vi "TTA_MATLAB_Load_Settings.vi"(0 "Instruments/Criteria Settings File":path, 5 "error in":errorcluster) -> (7 "Tx Output Power Criteria Cluster":T4, 8 "Complete Settings Cluster":T1, 9 "Rx Output Power Criteria Cluster":T2, 10 "TxOffset Cal Cluster":T10, 11 "Power Cal Cluster":T6, 12 "RxOffset Cal Cluster":T9, 13 "Tx ACPR Settings Cluster":T7, 14 "Brief Cluster":T13, 15 "PAL Calibration\nInputs Cluster":T11, 16 "TX Output Power Settings Cluster":T8, 17 "Rx Received Power Settings Cluster":T5, 18 "Instrument Setting Cluster":T12, 19 "error out":errorcluster)   [LabVIEW 2016]
uses:
  TTA_Controls/TTA_Control_Complete_Settings_Cluster.ctl
  TTA_Globals/Test_Environment.vi
panel:
  out "Tx ACPR Criteria Cluster":T3
  out "Error Range Cluster":cluster{dbl, dbl, dbl, dbl, dbl, dbl}
  out "Cal Turns Cluster":cluster{dbl, dbl, dbl, dbl, dbl}
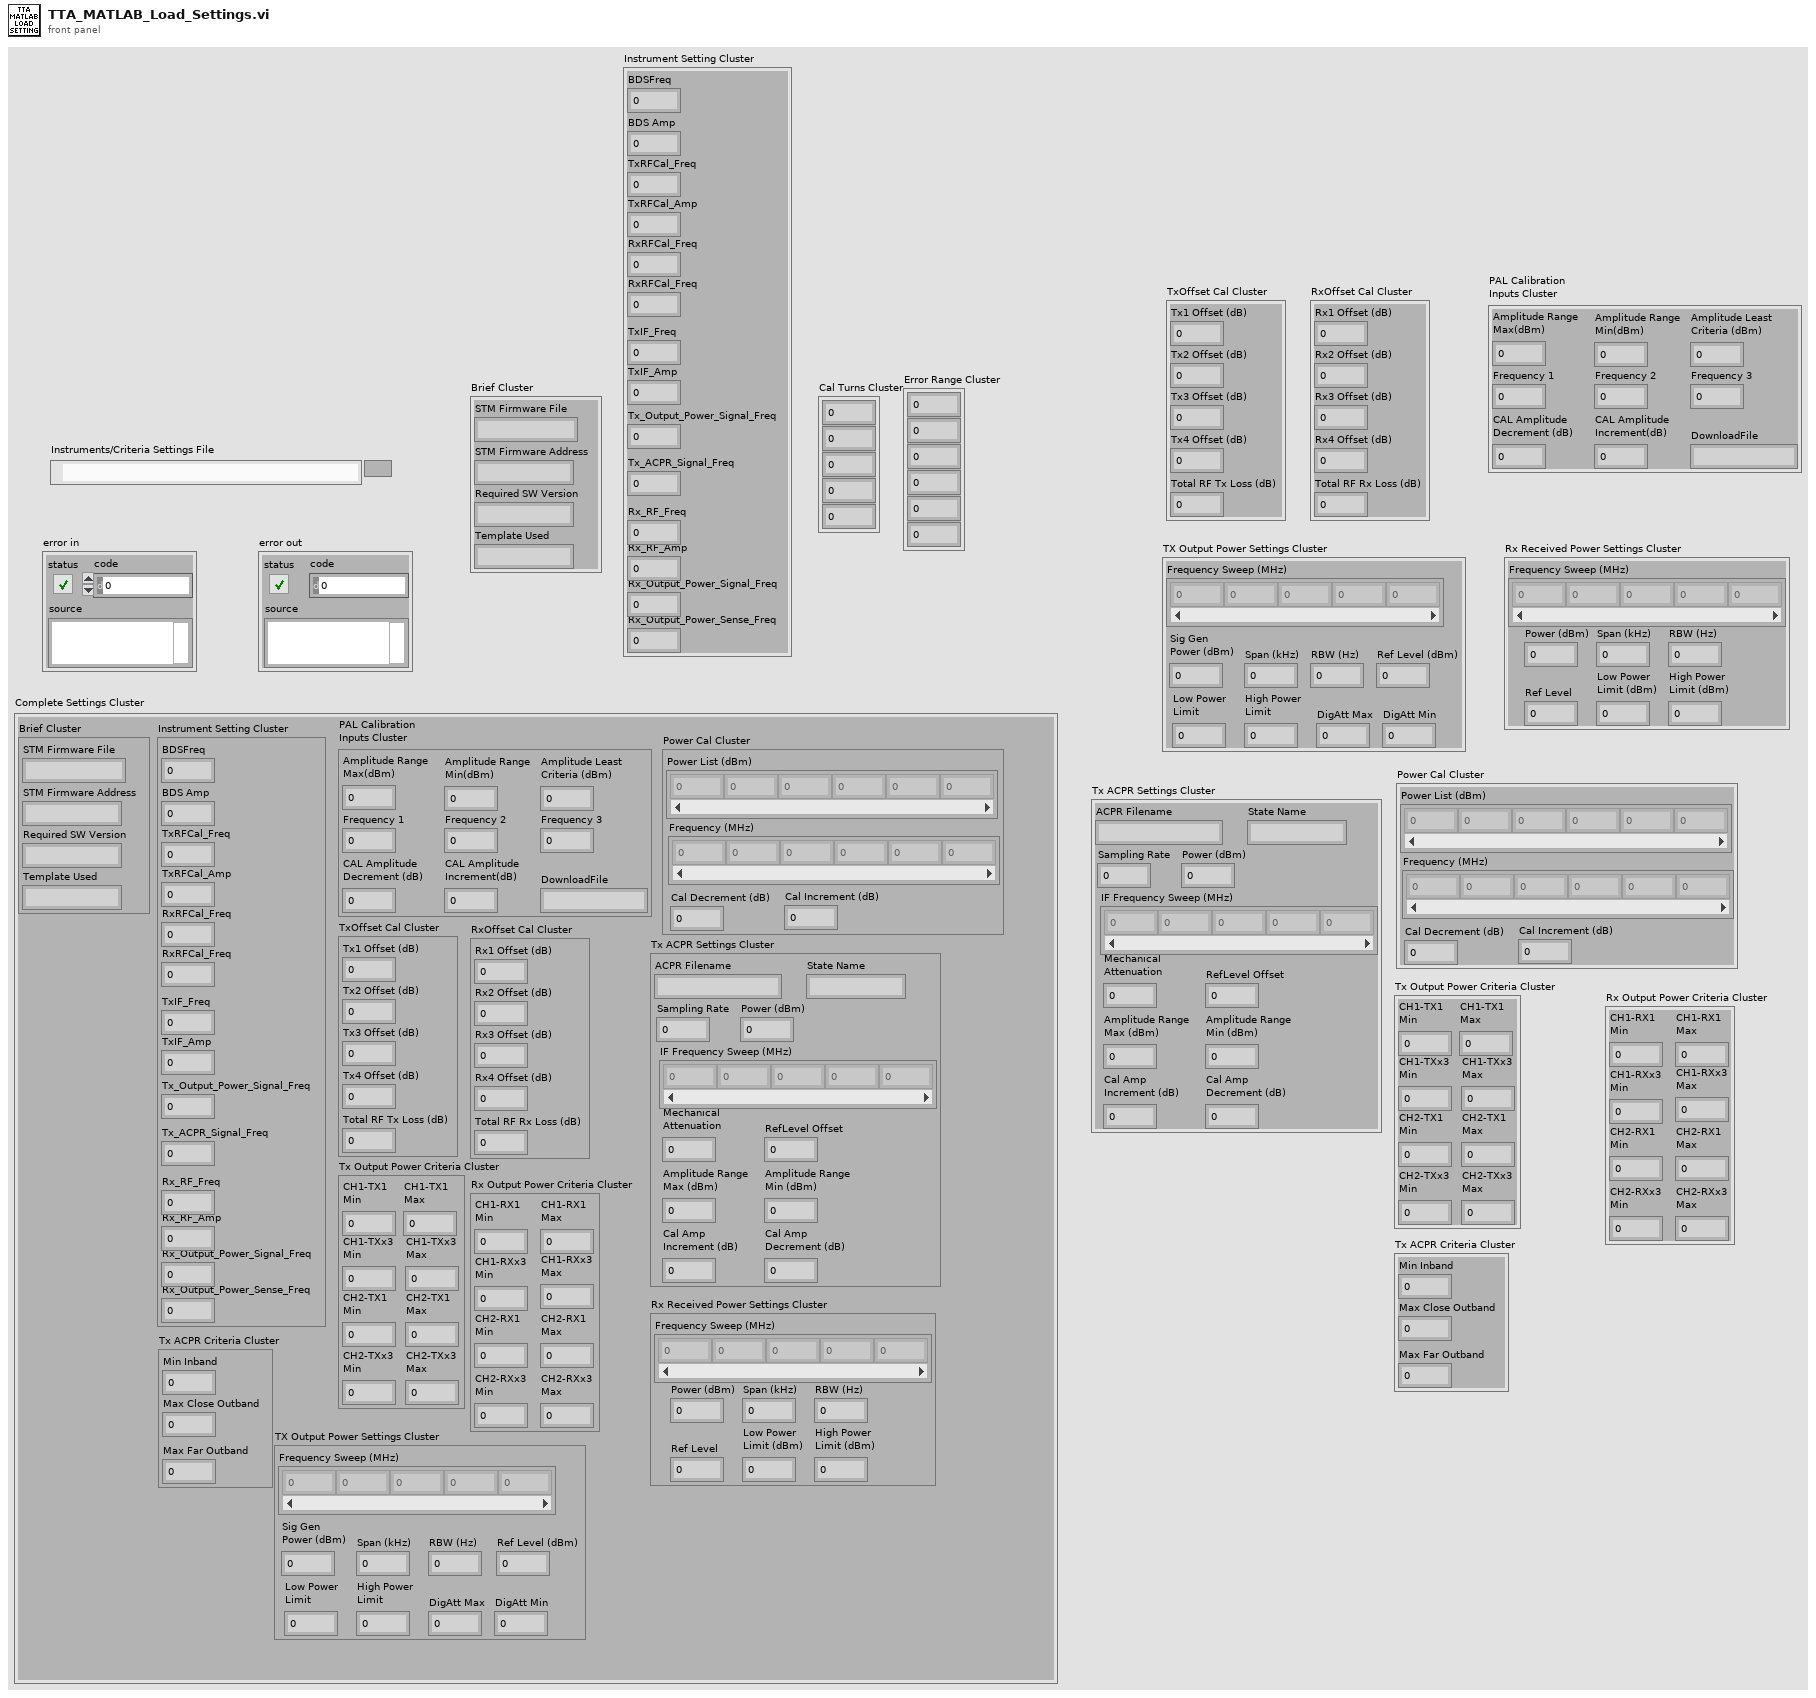
[diagram p1: front panel]
types:
  T1 = typedef "TTA_Control_Complete_Settings_Cluster.ctl" = cluster{"Brief Cluster":cluster{"STM Firmware File":string, "STM Firmware Address":string, "Required SW Version":string, "Template Used":string}, "Instrument Setting Cluster":cluster{"BDSFreq":dbl, "BDS Amp":dbl, "TxRFCal_Freq":dbl, "TxRFCal_Amp":dbl, "RxRFCal_Freq":dbl, "RxRFCal_Freq":dbl, "TxIF_Freq":dbl, "TxIF_Amp":dbl, "Tx_Output_Power_Signal_Freq":dbl, "Tx_ACPR_Signal_Freq":dbl, "Rx_RF_Freq":dbl, "Rx_RF_Amp":dbl, "Rx_Output_Power_Signal_Freq":dbl, "Rx_Output_Power_Sense_Freq":dbl}, "PAL Calibration\nInputs Cluster":cluster{"Amplitude Range\nMax(dBm)":dbl, "Amplitude Range\nMin(dBm)":dbl, "Amplitude Least\nCriteria (dBm)":dbl, "Frequency 1":dbl, "Frequency 2":dbl, "Frequency 3":dbl, "CAL Amplitude\nDecrement (dB)":dbl, "CAL Amplitude\nIncrement(dB)":dbl, "DownloadFile":string}, "TxOffset Cal Cluster":cluster{"Tx1 Offset (dB)":dbl, "Tx2 Offset (dB)":dbl, "Tx3 Offset (dB)":dbl, "Tx4 Offset (dB)":dbl, "Total RF Tx Loss (dB)":dbl}, "RxOffset Cal Cluster":cluster{"Rx1 Offset (dB)":dbl, "Rx2 Offset (dB)":dbl, "Rx3 Offset (dB)":dbl, "Rx4 Offset (dB)":dbl, "Total RF Rx Loss (dB)":dbl}, "TX Output Power Settings Cluster":cluster{"Frequency Sweep (MHz)":dbl[], "Sig Gen \nPower (dBm)":dbl, "Span (kHz)":dbl, "RBW (Hz)":dbl, "Ref Level (dBm)":dbl, "Low Power \nLimit":dbl, "High Power \nLimit":dbl, "DigAtt Max":dbl, "DigAtt Min":dbl}, "Tx ACPR Settings Cluster":cluster{"ACPR Filename":string, "Sampling Rate":dbl, "Power (dBm)":dbl, "IF Frequency Sweep (MHz)":dbl[], "State Name":string, "Mechanical\nAttenuation":dbl, "RefLevel Offset":dbl, "Amplitude Range\nMax (dBm)":dbl, "Amplitude Range\nMin (dBm)":dbl, "Cal Amp \nIncrement (dB)":dbl, "Cal Amp\nDecrement (dB)":dbl}, "Power Cal Cluster":cluster{"Power List (dBm)":dbl[], "Frequency (MHz)":dbl[], "Cal Decrement (dB)":dbl, "Cal Increment (dB)":dbl}, "Rx Received Power Settings Cluster":cluster{"Frequency Sweep (MHz)":dbl[], "Power (dBm)":dbl, "Span (kHz)":dbl, "RBW (Hz)":dbl, "Ref Level":dbl, "Low Power \nLimit (dBm)":dbl, "High Power\nLimit (dBm)":dbl}, "Tx Output Power Criteria Cluster":cluster{"CH1-TX1 \nMin":dbl, "CH1-TX1\nMax":dbl, "CH1-TXx3\nMin ":dbl, "CH1-TXx3\nMax":dbl, "CH2-TX1\nMin":dbl, "CH2-TX1\nMax":dbl, "CH2-TXx3\nMin":dbl, "CH2-TXx3\nMax":dbl}, "Tx ACPR Criteria Cluster":cluster{"Min Inband":dbl, "Max Close Outband":dbl, "Max Far Outband":dbl}, "Rx Output Power Criteria Cluster":cluster{"CH1-RX1 \nMin":dbl, "CH1-RX1 \nMax":dbl, "CH1-RXx3 \nMin":dbl, "CH1-RXx3\nMax":dbl, "CH2-RX1\nMin":dbl, "CH2-RX1\nMax":dbl, "CH2-RXx3\nMin":dbl, "CH2-RXx3\nMax":dbl}}
  T2 = cluster{"CH1-RX1 \nMin":dbl, "CH1-RX1 \nMax":dbl, "CH1-RXx3 \nMin":dbl, "CH1-RXx3\nMax":dbl, "CH2-RX1\nMin":dbl, "CH2-RX1\nMax":dbl, "CH2-RXx3\nMin":dbl, "CH2-RXx3\nMax":dbl}
  T3 = cluster{"Min Inband":dbl, "Max Close Outband":dbl, "Max Far Outband":dbl}
  T4 = cluster{"CH1-TX1 \nMin":dbl, "CH1-TX1\nMax":dbl, "CH1-TXx3\nMin ":dbl, "CH1-TXx3\nMax":dbl, "CH2-TX1\nMin":dbl, "CH2-TX1\nMax":dbl, "CH2-TXx3\nMin":dbl, "CH2-TXx3\nMax":dbl}
  T5 = cluster{"Frequency Sweep (MHz)":dbl[], "Power (dBm)":dbl, "Span (kHz)":dbl, "RBW (Hz)":dbl, "Ref Level":dbl, "Low Power \nLimit (dBm)":dbl, "High Power\nLimit (dBm)":dbl}
  T6 = cluster{"Power List (dBm)":dbl[], "Frequency (MHz)":dbl[], "Cal Decrement (dB)":dbl, "Cal Increment (dB)":dbl}
  T7 = cluster{"ACPR Filename":string, "Sampling Rate":dbl, "Power (dBm)":dbl, "IF Frequency Sweep (MHz)":dbl[], "State Name":string, "Mechanical\nAttenuation":dbl, "RefLevel Offset":dbl, "Amplitude Range\nMax (dBm)":dbl, "Amplitude Range\nMin (dBm)":dbl, "Cal Amp \nIncrement (dB)":dbl, "Cal Amp\nDecrement (dB)":dbl}
  T8 = cluster{"Frequency Sweep (MHz)":dbl[], "Sig Gen \nPower (dBm)":dbl, "Span (kHz)":dbl, "RBW (Hz)":dbl, "Ref Level (dBm)":dbl, "Low Power \nLimit":dbl, "High Power \nLimit":dbl, "DigAtt Max":dbl, "DigAtt Min":dbl}
  T9 = cluster{"Rx1 Offset (dB)":dbl, "Rx2 Offset (dB)":dbl, "Rx3 Offset (dB)":dbl, "Rx4 Offset (dB)":dbl, "Total RF Rx Loss (dB)":dbl}
  T10 = cluster{"Tx1 Offset (dB)":dbl, "Tx2 Offset (dB)":dbl, "Tx3 Offset (dB)":dbl, "Tx4 Offset (dB)":dbl, "Total RF Tx Loss (dB)":dbl}
  T11 = cluster{"Amplitude Range\nMax(dBm)":dbl, "Amplitude Range\nMin(dBm)":dbl, "Amplitude Least\nCriteria (dBm)":dbl, "Frequency 1":dbl, "Frequency 2":dbl, "Frequency 3":dbl, "CAL Amplitude\nDecrement (dB)":dbl, "CAL Amplitude\nIncrement(dB)":dbl, "DownloadFile":string}
  T12 = cluster{"BDSFreq":dbl, "BDS Amp":dbl, "TxRFCal_Freq":dbl, "TxRFCal_Amp":dbl, "RxRFCal_Freq":dbl, "RxRFCal_Freq":dbl, "TxIF_Freq":dbl, "TxIF_Amp":dbl, "Tx_Output_Power_Signal_Freq":dbl, "Tx_ACPR_Signal_Freq":dbl, "Rx_RF_Freq":dbl, "Rx_RF_Amp":dbl, "Rx_Output_Power_Signal_Freq":dbl, "Rx_Output_Power_Sense_Freq":dbl}
  T13 = cluster{"STM Firmware File":string, "STM Firmware Address":string, "Required SW Version":string, "Template Used":string}
  T14 = cluster{dbl, dbl, dbl, dbl, dbl, dbl, dbl, dbl, string}
  T15 = cluster{dbl[], dbl, dbl, dbl, dbl, dbl, dbl, dbl, dbl}
  T16 = cluster{string, dbl, dbl, dbl[], string, dbl, dbl, dbl, dbl, dbl, dbl}
  T17 = cluster{dbl, dbl, dbl, dbl, dbl, dbl, dbl, dbl, dbl, dbl, dbl, dbl, dbl, dbl}
  T18 = cluster{cluster{string, string, string, string}, cluster{dbl, dbl, dbl, dbl, dbl, dbl, dbl, dbl, dbl, dbl, dbl, dbl, dbl, dbl}, cluster{dbl, dbl, dbl, dbl, dbl, dbl, dbl, dbl, string}, cluster{dbl, dbl, dbl, dbl, dbl}, cluster{dbl, dbl, dbl, dbl, dbl}, cluster{dbl[], dbl, dbl, dbl, dbl, dbl, dbl, dbl, dbl}, cluster{string, dbl, dbl, dbl[], string, dbl, dbl, dbl, dbl, dbl, dbl}, cluster{dbl[], dbl[], dbl, dbl}, cluster{dbl[], dbl, dbl, dbl, dbl, dbl, dbl}, cluster{dbl, dbl, dbl, dbl, dbl, dbl, dbl, dbl}, cluster{dbl, dbl, dbl}, cluster{dbl, dbl, dbl, dbl, dbl, dbl, dbl, dbl}}
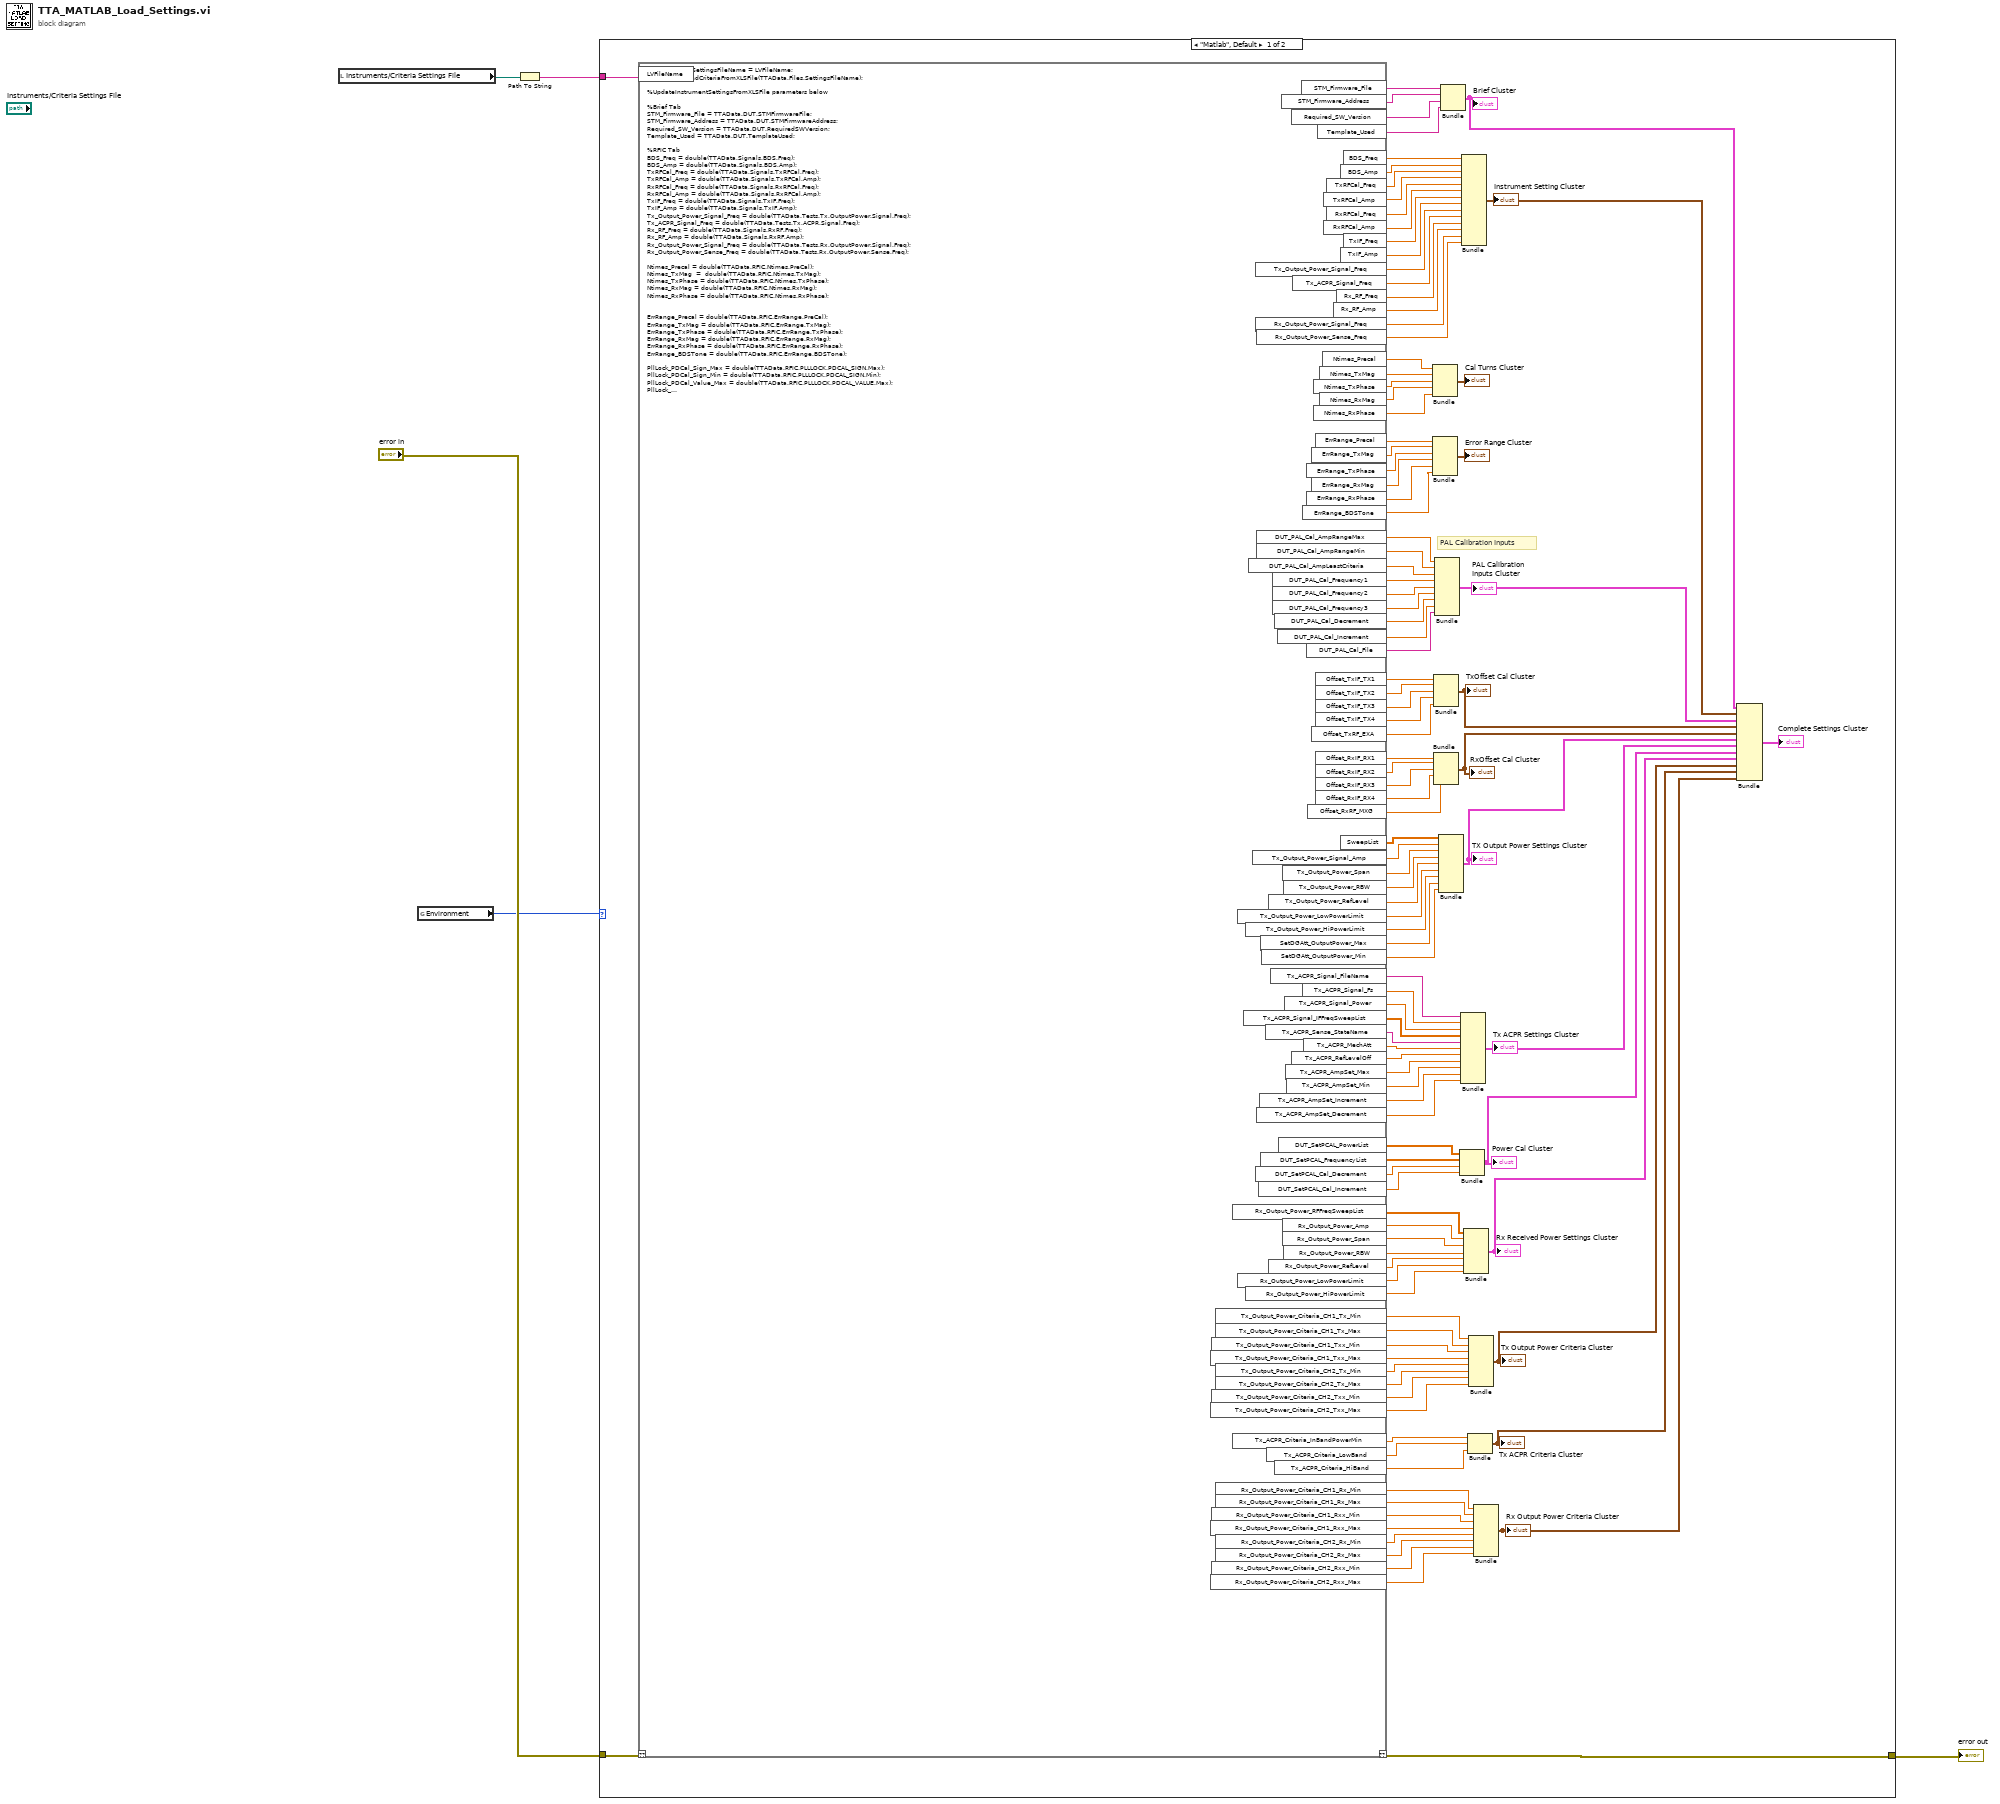
[diagram p0: block diagram]
diagram:
  n1 = local read "Instruments/Criteria Settings File"() -> (w5:path)
  n2 = global read "Test_Environment.vi" "Environment"() -> (w1:enum16{"Matlab", "LabVIEW"})
  n3 = Path To String(path=w5) -> (string=w4:string)
  n4 = case shown="\"Matlab\", Default" w1 {
    tunnel: w4 -> [w121 _]
    tunnel: "error in" -> [w120 w122]
    tunnel: [w119 w122] -> w2
    frame "Matlab", Default {
      # "PAL Calibration Inputs"
      n5 = script code="TTAData.Files.SettingsFileName = LVFileName;\nLoadSettingsAndCriteriaFromXLSFile(TTAData.Files.SettingsFileName);\n\n%UpdateInstrumentSettingsFromXLSFile parameters below\n\n%Brief Tab\nSTM_Firmware_File = TTAData.DUT.STMFirmwareFile;\nSTM_Firmware_Address = TTAData.DUT.STMFirmwareAddress;\nRequired_SW_Version = TTAData.DUT.RequiredSWVersion;\nTemplate_Used = TTAData.DUT.TemplateUsed;\n\n%RFIC Tab\nBDS_Freq = double(TTAData.Signals.BDS.Freq);\nBDS_Amp = double(TTAData.Signals.BDS.Amp);\nTxRFCal_Freq = double(TTAData.Signals.TxRFCal.Freq);\nTxRFCal_Amp = double(TTAData.Signals.TxRFCal.Amp);\nRxRFCal_Freq = double(TTAData.Signals.RxRFCal.Freq);\nRxRFCal_Amp = double(TTAData.Signals.RxRFCal.Amp);\nTxIF_Freq = double(TTAData.Signals.TxIF.Freq);\nTxIF_Amp = double(TTAData.Signals.TxIF.Amp);\nTx_Output_Power_Signal_Freq = double(TTAData.Tests.Tx.OutputPower.Signal.Freq);\nTx_ACPR_Signal_Freq = double(TTAData.Tests.Tx.ACPR.Signal.Freq);\nRx_RF_Freq = double(TTAData.Signals.RxRF.Freq);\nRx_RF_Amp = double(TTAData.Signals.RxRF.Amp);\nRx_Output_Power_Signal_Freq = double(TTAData.Tests.Rx.OutputPower.Signal.Freq);\nRx_Output_Power_Sense_Freq = double(TTAData.Tests.Rx.OutputPower.Sense.Freq);\n\nNtimes_Precal = double(TTAData.RFIC.Ntimes.PreCal);\nNtimes_TxMag  =  double(TTAData.RFIC.Ntimes.TxMag);\nNtimes_TxPhase = double(TTAData.RFIC.Ntimes.TxPhase);\nNtimes_RxMag = double(TTAData.RFIC.Ntimes.RxMag);\nNtimes_RxPhase = double(TTAData.RFIC.Ntimes.RxPhase);\n\n\nErrRange_Precal = double(TTAData.RFIC.ErrRange.PreCal);\nErrRange_TxMag = double(TTAData.RFIC.ErrRange.TxMag);\nErrRange_TxPhase = double(TTAData.RFIC.ErrRange.TxPhase);\nErrRange_RxMag = double(TTAData.RFIC.ErrRange.RxMag);\nErrRange_RxPhase = double(TTAData.RFIC.ErrRange.RxPhase);\nErrRange_BDSTone = double(TTAData.RFIC.ErrRange.BDSTone);\n\nPllLock_PDCal_Sign_Max = double(TTAData.RFIC.PLLLOCK.PDCAL_SIGN.Max); \nPllLock_PDCal_Sign_Min = double(TTAData.RFIC.PLLLOCK.PDCAL_SIGN.Min);\nPllLock_PDCal_Value_Max = double(TTAData.RFIC.PLLLOCK.PDCAL_VALUE.Max);\nPllLock_PDCal_Value_Min = double(TTAData.RFIC.PLLLOCK.PDCAL_VALUE.Min);\nPllLock_Bcal_Max = double(TTAData.RFIC.PLLLOCK.BCAL.Max);\nPllLock_Bcal_Min = double(TTAData.RFIC.PLLLOCK.BCAL.Min);\nRFCal_MagCal_Max = double(TTAData.RFIC.RFCAL.MAGCAL.Max);\nRFCal_MagCal_Min = double(TTAData.RFIC.RFCAL.MAGCAL.Min);\nRFCal_PhCal_Max = double(TTAData.RFIC.RFCAL.PHCAL.Max);\nRFCal_PhCal_Min = double(TTAData.RFIC.RFCAL.PHCAL.Min);\nRF_Cal_PreCal_PdCal_Sign_Max = double(TTAData.RFIC.RFCAL.PRECAL.PDCAL_SIGN.Max);\nRF_Cal_PreCal_PdCal_Sign_Min = double(TTAData.RFIC.RFCAL.PRECAL.PDCAL_SIGN.Min);\nRF_Cal_PreCal_PdCal_Value_Max = double(TTAData.RFIC.RFCAL.PRECAL.PDCAL_VALUE.Max);\nRF_Cal_PreCal_PdCal_Value_Min = double(TTAData.RFIC.RFCAL.PRECAL.PDCAL_VALUE.Min);\nRF_Cal_PllLock_BCal_Max = double(TTAData.RFIC.RFCAL.PLLLOCK.BCAL_Max);\nRF_Cal_PllLock_BCal_Min = double(TTAData.RFIC.RFCAL.PLLLOCK.BCAL_Min);\nRFIC_Temp_Max = double(TTAData.RFIC.TEMP.Max);\nRFIC_Temp_Min = double(TTAData.RFIC.TEMP.Min);\nRFIC_RFCal_Mode_CoarseOnly = double(TTAData.RFIC.RFCAL.MODE.COARSEONLY);\nRFIC_RFCal_Mode_ExtFineStop = double(TTAData.RFIC.RFCAL.MODE.EXTFINESTOP);\nRFIC_RFCal_Mode_Att = double(TTAData.RFIC.RFCAL.MODE.ATT);\nRFIC_RFCal_Mode_PreDist = double(TTAData.RFIC.RFCAL.MODE.PREDIST);\nRFIC_RFCal_Mode_Deg180Fix = double(TTAData.RFIC.RFCAL.MODE.DEG180FIX);\nRFIC_RFCal_Mode_PAOutPwrLoop = double(TTAData.RFIC.RFCAL.MODE.PAOUTPWRLOOP);\nRFIC_RFCal_Mode_PAInPwrLoop = double(TTAData.RFIC.RFCAL.MODE.PAINPWRLOOP);\nRFIC_RFCal_Mode_PABias_Loop = double(TTAData.RFIC.RFCAL.MODE.PABIASLOOP);\nRFIC_RFCal_Att_Temp_Nom = double(TTAData.RFIC.RFCAL.ATT.TEMP_NOM);\nRFIC_RFCal_Att_Slope = double(TTAData.RFIC.RFCAL.ATT.SLOPE);\nRFIC_RFCal_DelayFine = double(TTAData.RFIC.RFCAL.DELAYFINE);\nRFIC_RFCal_TxAmpGain = double(TTAData.RFIC.RFCAL.TXAMPGAIN);\nRFIC_RFCal_Nom_Offset_MagTx = double(TTAData.RFIC.RFCAL.NOM_OFFSET_MAGTX);\nRFIC_RFCal_RxAmpGain =     double(TTAData.RFIC.RFCAL.RXAMPGAIN);\n\nRFIC_RFCal_Delay_RxRFCal = double(TTAData.RFIC.RFCAL.DELAY_RxRFCAL);\n\nRFIC_Nom_Mag_Tx = double(TTAData.RFIC.NOM_MAG_TX);\nRFIC_Nom_Mag_Rx = double(TTAData.RFIC.NOM_MAG_RX);\nRFIC_MagLUT = double(TTAData.RFIC.MAGLUT);\nRFIC_PhLUT = double(TTAData.RFIC.PHLUT);\nRFIC_Resample = double(TTAData.RFIC.RESAMPLE);\nRFIC_RFCal_DelayCourse = double(TTAData.RFIC.RFCAL.DELAYCOARSE);\n\n%*****************Tx ACPR Tab**********************\nDUT_PAL_Cal_AmpRangeMax = double(TTAData.DUT.PAL_CAL.AmpRangeMax);\nDUT_PAL_Cal_AmpRangeMin = double(TTAData.DUT.PAL_CAL.AmpRangeMin);\nDUT_PAL_Cal_AmpLeastCriteria = double(TTAData.DUT.PAL_CAL.AmpLeastCriteria);\nDUT_PAL_Cal_Frequency1 = double(TTAData.DUT.PAL_CAL.Frequency1);\nDUT_PAL_Cal_Frequency2 = double(TTAData.DUT.PAL_CAL.Frequency2);\nDUT_PAL_Cal_Frequency3 = double(TTAData.DUT.PAL_CAL.Frequency3);\nDUT_PAL_Cal_Decrement = double(TTAData.DUT.PAL_CAL.CAL_Decrement);\nDUT_PAL_Cal_Increment = double(TTAData.DUT.PAL_CAL.CAL_Increment);\nDUT_PAL_Cal_File = char(TTAData.DUT.PAL_CAL.DownloadFile);\n\nTx_ACPR_Signal_FileName = char(TTAData.Tests.Tx.ACPR.Signal.FileName);\nTx_ACPR_Signal_Fs = double(TTAData.Tests.Tx.ACPR.Signal.Fs);\nTx_ACPR_Signal_Power = double(TTAData.Tests.Tx.ACPR.Signal.Power);\nTx_ACPR_Signal_IFFreqSweepList = double(TTAData.Tests.Tx.ACPR.Signal.IFFreqSweepList);\nTx_ACPR_Sense_StateName = char(TTAData.Tests.Tx.ACPR.Sense.StateName);\nTx_ACPR_MechAtt = double(TTAData.Tests.Tx.ACPR.MechAtt);\nTx_ACPR_RefLevelOff = double(TTAData.Tests.Tx.ACPR.RefLevelOff);\nTx_ACPR_AmpSet_Max = double(TTAData.Tests.Tx.ACPR.AmpSet.Max);\nTx_ACPR_AmpSet_Min = double(TTAData.Tests.Tx.ACPR.AmpSet.Min);\nTx_ACPR_AmpSet_Increment = double(TTAData.Tests.Tx.ACPR.AmpSet.Increment);\nTx_ACPR_AmpSet_Decrement = double(TTAData.Tests.Tx.ACPR.AmpSet.Decrement);\n\n%*****************TxRxOffset CAL Tab**********************\nOffset_TxIF_TX1 = double(TTAData.Offset.TxIF.TX1);\nOffset_TxIF_TX2 = double(TTAData.Offset.TxIF.TX2);\nOffset_TxIF_TX3 = double(TTAData.Offset.TxIF.TX3);\nOffset_TxIF_TX4 = double(TTAData.Offset.TxIF.TX4);\nOffset_TxIF_TXx3 = double(TTAData.Offset.TxIF.TXx3);\nOffset_TxIF_TXx4 = double(TTAData.Offset.TxIF.TXx4);\nOffset_TxRF_EXA = double(TTAData.Offset.TxRF.EXA);\n\nOffset_RxIF_RX1 = double(TTAData.Offset.RxIF.RX1);\nOffset_RxIF_RX2 = double(TTAData.Offset.RxIF.RX2);\nOffset_RxIF_RX3 = double(TTAData.Offset.RxIF.RX3);\nOffset_RxIF_RX4 = double(TTAData.Offset.RxIF.RX4);\nOffset_RxIF_RXx3 = double(TTAData.Offset.RxIF.RXx3);\nOffset_RxIF_RXx4 = double(TTAData.Offset.RxIF.RXx4);\nOffset_RxRF_MXG = double(TTAData.Offset.RxRF.MXG);\n\n%*****************Tx Output Power Tab**********************\nSweepList = double(TTAData.Tests.Tx.OutputPower.Signal.IFFreqSweepList);\nTx_Output_Power_Signal_Amp = double(TTAData.Tests.Tx.OutputPower.Signal.Amp);;\nTx_Output_Power_Span = double(TTAData.Tests.Tx.OutputPower.Sense.Span);\nTx_Output_Power_RBW = double(TTAData.Tests.Tx.OutputPower.Sense.RBW);\nTx_Output_Power_RefLevel = double(TTAData.Tests.Tx.OutputPower.Sense.RefLevel);\nTx_Output_Power_LowPowerLimit= double(TTAData.Tests.Tx.OutputPower.Sense.LowPowerLimit);\nTx_Output_Power_HiPowerLimit = double(TTAData.Tests.Tx.OutputPower.Sense.HiPowerLimit);\nSetDGAtt_OutputPower_Max = double(TTAData.SetDGAtt.OutputPower.Max);\nSetDGAtt_OutputPower_Min = double(TTAData.SetDGAtt.OutputPower.Min);\n\n%*****************Power Cal Tab**********************\nDUT_SetPCAL_PowerList = double(TTAData.DUT.SetPCAL.PowerList);\nDUT_SetPCAL_FrequencyList = double(TTAData.DUT.SetPCAL.Frequency);\nDUT_SetPCAL_Cal_Decrement = double(TTAData.DUT.SetPCAL.CAL_Decrement);\nDUT_SetPCAL_Cal_Increment = double(TTAData.DUT.SetPCAL.CAL_Increment);\n\n%*****************Rx Received Power Tab**********************\nRx_Output_Power_RFFreqSweepList = double(TTAData.Tests.Rx.OutputPower.Signal.RFFreqSweepList);\nRx_Output_Power_Amp = double(TTAData.Tests.Rx.OutputPower.Signal.Amp);\nRx_Output_Power_Span = double(TTAData.Tests.Rx.OutputPower.Sense.Span);\nRx_Output_Power_RBW = double(TTAData.Tests.Rx.OutputPower.Sense.RBW);\nRx_Output_Power_RefLevel = double(TTAData.Tests.Rx.OutputPower.Sense.RefLevel);\nRx_Output_Power_LowPowerLimit = double(TTAData.Tests.Rx.OutputPower.Sense.LowPowerLimit);\nRx_Output_Power_HiPowerLimit = double(TTAData.Tests.Rx.OutputPower.Sense.HiPowerLimit);\n\n\n%*****************Tx Output Power Criteria**********************\nTx_Output_Power_Criteria_CH1_Tx_Min = double(TTAData.Tests.Tx.OutputPower.Criteria.CH1Tx.MinIFAmp);\nTx_Output_Power_Criteria_CH1_Tx_Max = double(TTAData.Tests.Tx.OutputPower.Criteria.CH1Tx.MaxIFAmp);\nTx_Output_Power_Criteria_CH1_Txx_Min = double(TTAData.Tests.Tx.OutputPower.Criteria.CH1Txx.MinIFAmp);\nTx_Output_Power_Criteria_CH1_Txx_Max = double(TTAData.Tests.Tx.OutputPower.Criteria.CH1Txx.MaxIFAmp);\nTx_Output_Power_Criteria_CH2_Tx_Min = double(TTAData.Tests.Tx.OutputPower.Criteria.CH2Tx.MinIFAmp);\nTx_Output_Power_Criteria_CH2_Tx_Max = double(TTAData.Tests.Tx.OutputPower.Criteria.CH2Tx.MaxIFAmp);\nTx_Output_Power_Criteria_CH2_Txx_Min = double(TTAData.Tests.Tx.OutputPower.Criteria.CH2Txx.MinIFAmp);\nTx_Output_Power_Criteria_CH2_Txx_Max = double(TTAData.Tests.Tx.OutputPower.Criteria.CH2Txx.MaxIFAmp);\n\n%*****************Tx ACPR Criteria**********************\nTx_ACPR_Criteria_InBandPowerMin = double(TTAData.Tests.Tx.ACPR.Criteria.InBandPowerMin);\nTx_ACPR_Criteria_LowBand = double(TTAData.Tests.Tx.ACPR.Criteria.ACPRLowBand);\nTx_ACPR_Criteria_HiBand = double(TTAData.Tests.Tx.ACPR.Criteria.ACPRHiBand);\n\n%*****************Rx Received Power Criteria**********************\nRx_Output_Power_Criteria_CH1_Rx_Min = double(TTAData.Tests.Rx.OutputPower.Criteria.CH1Rx.MinIFAmp);\nRx_Output_Power_Criteria_CH1_Rx_Max = double(TTAData.Tests.Rx.OutputPower.Criteria.CH1Rx.MaxIFAmp);\nRx_Output_Power_Criteria_CH1_Rxx_Min = double(TTAData.Tests.Rx.OutputPower.Criteria.CH1Rxx.MinIFAmp);\nRx_Output_Power_Criteria_CH1_Rxx_Max = double(TTAData.Tests.Rx.OutputPower.Criteria.CH1Rxx.MaxIFAmp);\nRx_Output_Power_Criteria_CH2_Rx_Min = double(TTAData.Tests.Rx.OutputPower.Criteria.CH2Rx.MinIFAmp);\nRx_Output_Power_Criteria_CH2_Rx_Max = double(TTAData.Tests.Rx.OutputPower.Criteria.CH2Rx.MaxIFAmp);\nRx_Output_Power_Criteria_CH2_Rxx_Min = double(TTAData.Tests.Rx.OutputPower.Criteria.CH2Rxx.MinIFAmp);\nRx_Output_Power_Criteria_CH2_Rxx_Max = double(TTAData.Tests.Rx.OutputPower.Criteria.CH2Rxx.MaxIFAmp);"("??"=w120, "LVFileName"=w121) -> ("??"=w119:errorcluster, "STM_Firmware_File"=w118:string, "STM_Firmware_Address"=w117:string, "Required_SW_Version"=w116:string, "Template_Used"=w115:string, "BDS_Freq"=w108:dbl, "BDS_Amp"=w107:dbl, "TxRFCal_Freq"=w106:dbl, "TxRFCal_Amp"=w105:dbl, "RxRFCal_Freq"=w104:dbl, "RxRFCal_Amp"=w103:dbl, "TxIF_Freq"=w102:dbl, "TxIF_Amp"=w101:dbl, "Tx_Output_Power_Signal_Freq"=w100:dbl, "Tx_ACPR_Signal_Freq"=w99:dbl, "Rx_RF_Freq"=w98:dbl, "Rx_RF_Amp"=w97:dbl, "Rx_Output_Power_Signal_Freq"=w96:dbl, "Rx_Output_Power_Sense_Freq"=w95:dbl, "Ntimes_Precal"=w114:dbl, "Ntimes_TxMag"=w113:dbl, "Ntimes_TxPhase"=w112:dbl, "Ntimes_RxMag"=w111:dbl, "Ntimes_RxPhase"=w110:dbl, "ErrRange_Precal"=w94:dbl, "ErrRange_TxMag"=w93:dbl, "ErrRange_TxPhase"=w92:dbl, "ErrRange_RxMag"=w91:dbl, "ErrRange_RxPhase"=w90:dbl, "ErrRange_BDSTone"=w89:dbl, "DUT_PAL_Cal_AmpRangeMax"=w87:dbl, "DUT_PAL_Cal_AmpRangeMin"=w86:dbl, "DUT_PAL_Cal_AmpLeastCriteria"=w85:dbl, "DUT_PAL_Cal_Frequency1"=w84:dbl, "DUT_PAL_Cal_Frequency2"=w83:dbl, "DUT_PAL_Cal_Frequency3"=w82:dbl, "DUT_PAL_Cal_Decrement"=w81:dbl, "DUT_PAL_Cal_Increment"=w80:dbl, "DUT_PAL_Cal_File"=w79:string, "Offset_TxIF_TX1"=w78:dbl, "Offset_TxIF_TX2"=w77:dbl, "Offset_TxIF_TX3"=w76:dbl, "Offset_TxIF_TX4"=w75:dbl, "Offset_TxRF_EXA"=w74:dbl, "Offset_RxIF_RX1"=w73:dbl, "Offset_RxIF_RX2"=w72:dbl, "Offset_RxIF_RX3"=w71:dbl, "Offset_RxIF_RX4"=w70:dbl, "Offset_RxRF_MXG"=w69:dbl, "SweepList"=w7:dbl[], "Tx_Output_Power_Signal_Amp"=w8:dbl, "Tx_Output_Power_Span"=w68:dbl, "Tx_Output_Power_RBW"=w67:dbl, "Tx_Output_Power_RefLevel"=w66:dbl, "Tx_Output_Power_LowPowerLimit"=w65:dbl, "Tx_Output_Power_HiPowerLimit"=w64:dbl, "SetDGAtt_OutputPower_Max"=w63:dbl, "SetDGAtt_OutputPower_Min"=w62:dbl, "Tx_ACPR_Signal_FileName"=w51:string, "Tx_ACPR_Signal_Fs"=w52:dbl, "Tx_ACPR_Signal_Power"=w53:dbl, "Tx_ACPR_Signal_IFFreqSweepList"=w61:dbl[], "Tx_ACPR_Sense_StateName"=w60:string, "Tx_ACPR_MechAtt"=w59:dbl, "Tx_ACPR_RefLevelOff"=w58:dbl, "Tx_ACPR_AmpSet_Max"=w57:dbl, "Tx_ACPR_AmpSet_Min"=w56:dbl, "Tx_ACPR_AmpSet_Increment"=w55:dbl, "Tx_ACPR_AmpSet_Decrement"=w54:dbl, "DUT_SetPCAL_PowerList"=w50:dbl[], "DUT_SetPCAL_FrequencyList"=w49:dbl[], "DUT_SetPCAL_Cal_Decrement"=w48:dbl, "DUT_SetPCAL_Cal_Increment"=w47:dbl, "Rx_Output_Power_RFFreqSweepList"=w46:dbl[], "Rx_Output_Power_Amp"=w45:dbl, "Rx_Output_Power_Span"=w44:dbl, "Rx_Output_Power_RBW"=w43:dbl, "Rx_Output_Power_RefLevel"=w42:dbl, "Rx_Output_Power_LowPowerLimit"=w41:dbl, "Rx_Output_Power_HiPowerLimit"=w40:dbl, "Tx_Output_Power_Criteria_CH1_Tx_Min"=w39:dbl, "Tx_Output_Power_Criteria_CH1_Tx_Max"=w38:dbl, "Tx_Output_Power_Criteria_CH1_Txx_Min"=w37:dbl, "Tx_Output_Power_Criteria_CH1_Txx_Max"=w36:dbl, "Tx_Output_Power_Criteria_CH2_Tx_Min"=w35:dbl, "Tx_Output_Power_Criteria_CH2_Tx_Max"=w34:dbl, "Tx_Output_Power_Criteria_CH2_Txx_Min"=w33:dbl, "Tx_Output_Power_Criteria_CH2_Txx_Max"=w32:dbl, "Tx_ACPR_Criteria_InBandPowerMin"=w31:dbl, "Tx_ACPR_Criteria_LowBand"=w30:dbl, "Tx_ACPR_Criteria_HiBand"=w29:dbl, "Rx_Output_Power_Criteria_CH1_Rx_Min"=w28:dbl, "Rx_Output_Power_Criteria_CH1_Rx_Max"=w27:dbl, "Rx_Output_Power_Criteria_CH1_Rxx_Min"=w26:dbl, "Rx_Output_Power_Criteria_CH1_Rxx_Max"=w25:dbl, "Rx_Output_Power_Criteria_CH2_Rx_Min"=w24:dbl, "Rx_Output_Power_Criteria_CH2_Rx_Max"=w23:dbl, "Rx_Output_Power_Criteria_CH2_Rxx_Min"=w22:dbl, "Rx_Output_Power_Criteria_CH2_Rxx_Max"=w21:dbl)
      n6 = Bundle(w114, w113, w112, w111, w110) -> (→"Cal Turns Cluster":cluster{dbl, dbl, dbl, dbl, dbl})  [unwired: 1 in]
      n7 = Bundle(w94, w93, w92, w91, w90, w89) -> (→"Error Range Cluster":cluster{dbl, dbl, dbl, dbl, dbl, dbl})  [unwired: 1 in]
      n8 = Bundle(w78, w77, w76, w75, w74) -> (w17:cluster{dbl, dbl, dbl, dbl, dbl})  [unwired: 1 in]
      "TxOffset Cal Cluster" <- w17
      n9 = Bundle(w73, w72, w71, w70, w69) -> (w16:cluster{dbl, dbl, dbl, dbl, dbl})  [unwired: 1 in]
      "RxOffset Cal Cluster" <- w16
      n10 = Bundle(w87, w86, w85, w84, w83, w82, w81, w80, w79) -> (w18:T14)  [unwired: 1 in]
      "PAL Calibration\nInputs Cluster" <- w18
      n11 = Bundle(w7, w8, w68, w67, w66, w65, w64, w63, w62) -> (w6:T15)  [unwired: 1 in]
      "TX Output Power Settings Cluster" <- w6
      n12 = Bundle(w118, w117, w116, w115) -> (w20:cluster{string, string, string, string})  [unwired: 1 in]
      "Brief Cluster" <- w20
      n13 = Bundle(w50, w49, w48, w47) -> (w14:cluster{dbl[], dbl[], dbl, dbl})  [unwired: 1 in]
      "Power Cal Cluster" <- w14
      n14 = Bundle(w51, w52, w53, w61, w60, w59, w58, w57, w56, w55, w54) -> (w15:T16)  [unwired: 1 in]
      "Tx ACPR Settings Cluster" <- w15
      n15 = Bundle(w108, w107, w106, w105, w104, w103, w102, w101, w100, w99, w98, w97, w96, w95) -> (w19:T17)  [unwired: 1 in]
      "Instrument Setting Cluster" <- w19
      n16 = Bundle(w46, w45, w44, w43, w42, w41, w40) -> (w13:cluster{dbl[], dbl, dbl, dbl, dbl, dbl, dbl})  [unwired: 1 in]
      "Rx Received Power Settings Cluster" <- w13
      n17 = Bundle(w31, w30, w29) -> (w11:cluster{dbl, dbl, dbl})  [unwired: 1 in]
      "Tx ACPR Criteria Cluster" <- w11
      n18 = Bundle(w39, w38, w37, w36, w35, w34, w33, w32) -> (w12:cluster{dbl, dbl, dbl, dbl, dbl, dbl, dbl, dbl})  [unwired: 1 in]
      "Tx Output Power Criteria Cluster" <- w12
      n19 = Bundle(w28, w27, w26, w25, w24, w23, w22, w21) -> (w10:cluster{dbl, dbl, dbl, dbl, dbl, dbl, dbl, dbl})  [unwired: 1 in]
      "Rx Output Power Criteria Cluster" <- w10
      n20 = Bundle(w20, w19, w18, w17, w16, w6, w15, w14, w13, w12, w11, w10) -> (→"Complete Settings Cluster":T18)  [unwired: 1 in]
    }
    frame "LabVIEW" {
    }
  }
  "error out" <- w2
